vi "Update Addon To Latest Version.vi"(8 "error in (no error)":errorcluster, 11 "Device Item Ref in":T1 format="%.0x") -> (0 "error out":errorcluster, 3 "Device Item Ref out":T1 format="%.0x")   [LabVIEW 2020, in "Instrument Addon Shared.lvlib"]
uses:
  Instrument Addon Shared.lvlib
  <vilib>/NI VeriStand/Custom Device API/Custom Device Item Ref.ctl
  <vilib>/NI VeriStand/Custom Device API/Custom Device Channel.ctl
  <vilib>/NI VeriStand/Custom Device API/Custom Device Channel Type.ctl
  NationalInstruments.VeriStand.SystemDefinitionAPI
  Constants.vi
  <vilib>/NI/NI VeriStand Advanced SysDef API/_SubVIs/SysDef.Search.GUIDs.vi
  <vilib>/NI VeriStand/Custom Device API/Custom Device API.lvlib
  <vilib>/NI/NI VeriStand Advanced SysDef API/SysDef API/Advanced System Definition.lvlib
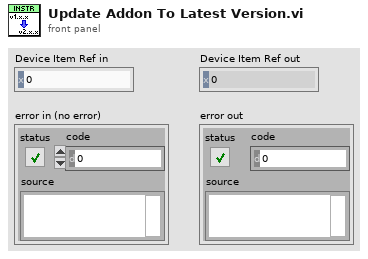
[diagram p1: front panel]
types:
  T1 = typedef "Custom Device API.lvlib/Custom Device Item Ref.ctl" = u64
  T2 = typedef "Custom Device API.lvlib/Custom Device Channel.ctl" = cluster{"Type":T3, "Units":string, "Default Value":dbl, "Faultable":bool, "Scalable":bool}
  T3 = typedef "Custom Device API.lvlib/Custom Device Channel Type.ctl" = enum16{"Input", "Output"}
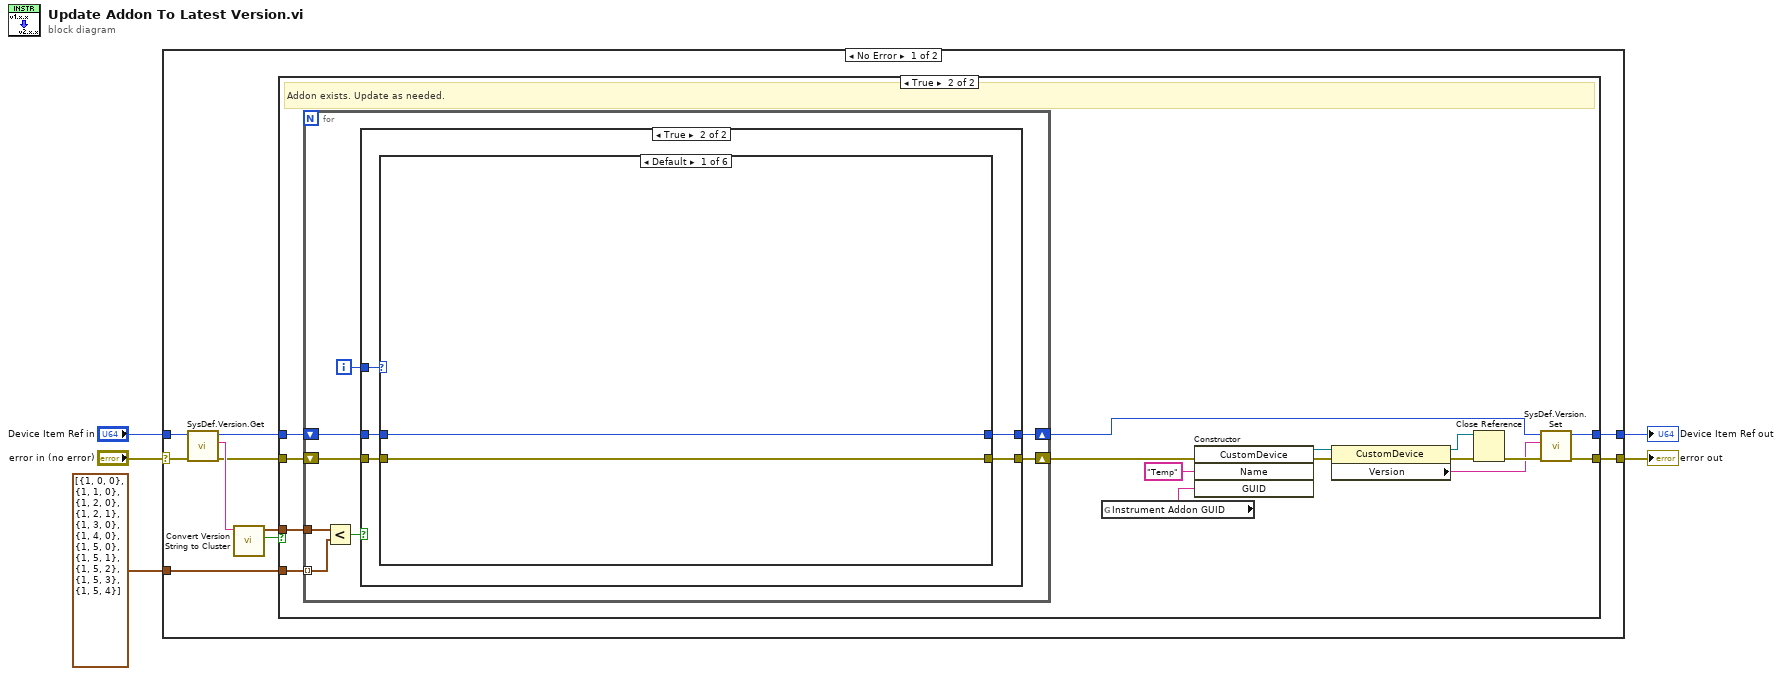
[diagram p0: block diagram]
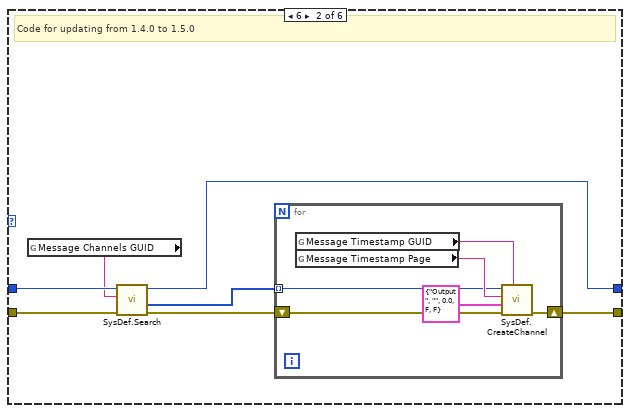
[diagram p4: hidden frame]
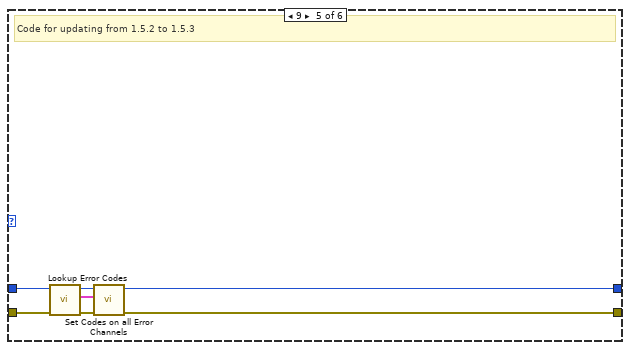
[diagram p7: hidden frame]
diagram:
  n1 = case shown="No Error" "error in (no error)" {
    selector: "error in (no error)" -> [w11 w78]
    tunnel: [w13 w78] -> w4
    tunnel: "Device Item Ref in" -> [w10 w77]
    tunnel: [w14 w77] -> w5
    tunnel: cluster{i32, i32, i32}[] [{1, 0, 0}, {1, 1, 0}, {1, 2, 0}, {1, 2, 1}, {1, 3, 0}, {1, 4, 0}, {1, 5, 0}, {1, 5, 1}, {1, 5, 2}, {1, 5, 3}, {1, 5, 4}] -> [w15 _]
    frame No Error {
      n2 = call <vilib>:"SysDef.Version.Get.vi"("error in (no error)"=w11, "nodeID"=w10) -> ("error out"=w9:errorcluster, "Version"=w12:string, "nodeID out"=w8:u64)  [unwired: 7 in]
      n3 = call "Convert Version String to Cluster.vi"("Version"=w12) -> ("Version Valid?"=w6:bool, "Version"=w7:cluster{i32, i32, i32})  [unwired: 9 in]
      n4 = case shown="True" w6 {
        tunnel: w15 -> [_ w33]
        tunnel: [w16 w26] -> w14
        tunnel: [w17 w25] -> w13
        tunnel: w7 -> [_ w20]
        tunnel: w9 -> [w17 w19]
        tunnel: w8 -> [w16 w18]
        frame False {
          # "Addon likely doesn't exist. Version not valid. Ignore."
        }
        frame True {
          # "Addon exists. Update as needed."
          n5 = for {
            shift-right: [w40] -> w24
            shift-left: w19 -> [w35]
            shift-right: [w39] -> w23
            shift-left: w18 -> [w34]
            tunnel: w33 -> [w36] mode=indexing
            tunnel: w20 -> [w37]
            i -> [w38]
            n6 = Less?(x=w37, y=w36) -> (x < y?=w41:bool)
            n7 = case shown="True" w41 {
              tunnel: w35 -> [w43 w48]
              tunnel: [w43 w47] -> w40
              tunnel: w34 -> [w42 w44]
              tunnel: [w42 w45] -> w39
              tunnel: w38 -> [_ w46]
              frame False {
              }
              frame True {
                n8 = case shown="Default" w46 {
                  tunnel: w48 -> [w50 w56 w65 w67 w70 w75]
                  tunnel: [w50 w51 w65 w67 w74 w75] -> w47
                  tunnel: [w49 w52 w64 w66 w73 w76] -> w45
                  tunnel: w44 -> [w49 w57 w64 w66 w72 w76]
                  frame Default {
                  }
                  frame 6 {
                    # "Code for updating from 1.4.0 to 1.5.0"
                    n9 = global read "Constants.vi" "Message Channels GUID"() -> (w55:string)
                    n10 = call-poly <vilib>:"SysDef.Search.vi"("error in (no error)"=w56, "GUID"=w55, "nodeID"=w57) -> ("error out"=w54:errorcluster, "Values Out"=w53:u64[], "nodeID out"=w52:u64)  [unwired: 5 in, 1 out]
                    n11 = for {
                      tunnel: w53 -> [w58] mode=indexing
                      shift-right: [w59] -> w51
                      shift-left: w54 -> [w60]
                      n12 = global read "Constants.vi" "Message Timestamp GUID"() -> (w62:string)
                      n13 = global read "Constants.vi" "Message Timestamp Page"() -> (w63:string)
                      n14 = call <vilib>:"SysDef.CreateChannel.vi"("GUID"=w62, "error in (no error)"=w60, "Channel"=T2 {"Type"=enum."Output", "Units"="", "Default Value"=0.0, "Faultable"=FALSE, "Scalable"=FALSE}, "Name"=w63, "nodeID"=w58) -> ("error out"=w59:errorcluster)  [unwired: 3 in, 3 out]
                    }
                  }
                  frame 7 {
                    # "Code for updating from 1.5.0 to 1.5.1"
                  }
                  frame 8 {
                    # "Code for updating from 1.5.1 to 1.5.2"
                  }
                  frame 9 {
                    # "Code for updating from 1.5.2 to 1.5.3"
                    n15 = call "Lookup Error Codes.vi"("error in (no error)"=w70, "Node Ptr"=w72) -> ("error out"=w69:errorcluster, "Error Codes"=w68:cluster{"Code":i32, "String":string}[], "Node Ptr out"=w71:u64)  [unwired: 7 in]
                    n16 = call "Set Codes on all Error Channels.vi"("error in (no error)"=w69, "Error Codes"=w68, "Node Ptr in"=w71) -> ("error out"=w74:errorcluster, "Section Ref out"=w73:T1)  [unwired: 7 in]
                  }
                  frame 10 {
                    # "Code for updating from 1.5.3 to 1.5.4"
                  }
                }
              }
            }
          }
          n17 = global read "Constants.vi" "Instrument Addon GUID"() -> (w21:string)
          n18 = constructor class="CustomDevice"(error in=w24, "Name"="Temp", "GUID"=w21) -> (reference out=w32:refnum<k24>, error out=w31:errorcluster)  [unwired: 2 in, 3 out]
          n19 = property class="CustomDevice"(reference=w32, error in=w31) -> (reference out=w29:refnum<k24>, error out=w30:errorcluster, "Version"=w27:string)
          n20 = Close Reference(reference=w29, error in (no error)=w30) -> (error out=w28:errorcluster)
          n21 = call <vilib>:"SysDef.Version.Set.vi"("error in (no error)"=w28, "Version"=w27, "nodeID"=w23) -> ("error out"=w25:errorcluster, "nodeID out"=w26:u64)  [unwired: 7 in]
        }
      }
    }
    frame Error {
    }
  }
  "Device Item Ref out" <- w5
  "error out" <- w4
